vi "gun_turret_angle_control.vi"(8 "Reset Integral":bool, 9 "Sensor":dbl, 10 "Setpoint":dbl) -> (3 "Motor Power":dbl)   [LabVIEW 2011]
panel:
  in  "PID Const":cluster{"kP":dbl, "kI":dbl, "kD":dbl}
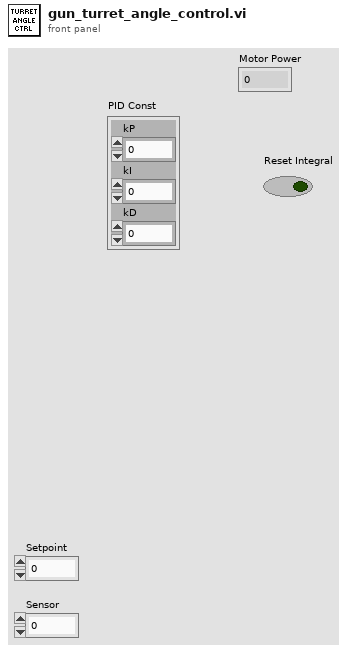
[diagram p1: front panel]
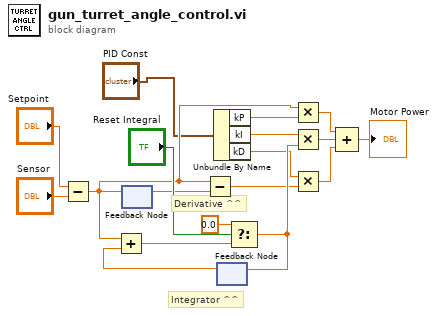
[diagram p0: block diagram]
diagram:
  # "Derivative ^^"
  # "Integrator ^^"
  n1 = Subtract(x="Setpoint", y="Sensor") -> (x-y=w5:dbl)
  n2 = feedback-in #1(w5) -> ()
  n3 = feedback #1() -> (w6:dbl)  [unwired: 1 in]
  n4 = Subtract(x=w5, y=w6) -> (x-y=w4:dbl)
  n5 = Unbundle By Name("PID Const") -> ("kP"=w16:dbl, "kI"=w7:dbl, "kD"=w3:dbl)
  n6 = feedback #2() -> (w13:dbl)  [unwired: 1 in]
  n7 = Add(x=w5, y=w13) -> (x+y=w12:dbl)
  n8 = Select(t=0.0, s="Reset Integral", f=w12) -> (s? t:f=w8:dbl)
  n9 = feedback-in #2(w8) -> ()
  n10 = Multiply(x=w5, y=w16) -> (x*y=w15:dbl)
  n11 = Multiply(x=w7, y=w8) -> (x*y=w9:dbl)
  n12 = Multiply(x=w3, y=w4) -> (x*y=w2:dbl)
  n13 = Compound Arithmetic op=ADD(w15, w9, w2) -> (→"Motor Power":dbl)
